vi "Add Destination.vi"(8 "error in (no error)":errorcluster, 9 "Destination type (directory)":T1, 10 "Destination label":string, 11 "EXE in":refnum<class "NI_AB_API_EXE.lvclass">) -> (0 "error out":errorcluster, 3 "EXE out":refnum<class "NI_AB_API_EXE.lvclass">)   [LabVIEW 2020, in "NI_AB_API_EXE.lvclass"]
uses:
  <vilib>/AppBuilder/AB_API/EXE/NI_AB_API_EXE.lvclass
  <vilib>/AppBuilder/AB_API/common/AB_API Destination Type.ctl
  <vilib>/AppBuilder/AB_API/Application/NI_AB_API_Application.lvclass
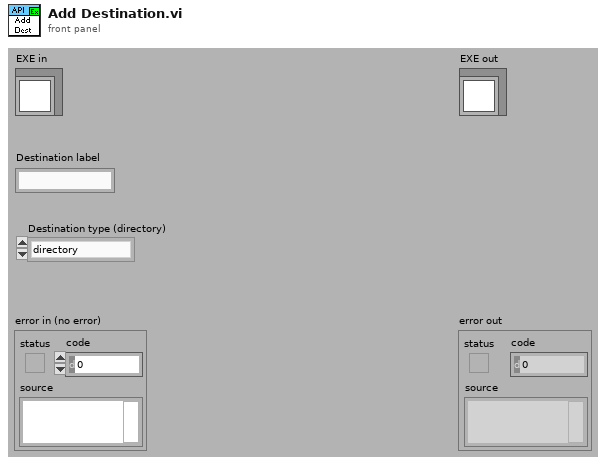
[diagram p1: front panel]
types:
  T1 = typedef "AB_API Destination Type.ctl" = enum16{"directory", "directory (preserve hierarchy)", "LLB"}
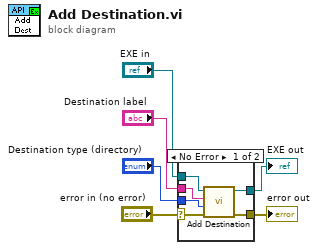
[diagram p0: block diagram]
diagram:
  n1 = case shown="No Error" "error in (no error)" {
    selector: "error in (no error)" -> [w10 w14]
    tunnel: [w9 w14] -> w4
    tunnel: [w11 w13] -> w5
    tunnel: "EXE in" -> [w12 w13]
    tunnel: "Destination label" -> [w8 _]
    tunnel: "Destination type (directory)" -> [w7 _]
    frame No Error {
      n2 = call-parent "Add Destination.vi"("error in (no error)"=w10, "Destination type (directory)"=w7, "Destination label"=w8, "Build in"=w12) -> ("error out"=w9:errorcluster, "Build out"=w11:refnum<class "NI_AB_API_EXE.lvclass">)  [unwired: 6 in]
    }
    frame Error {
    }
  }
  "error out" <- w4
  "EXE out" <- w5
